vi "5492_Get_YPRHfH.vi"(5 "Device Number":T1, 7 "Update":bool, 8 "error in":errorcluster) -> (0 "error out":errorcluster, 2 "YRPHfH":T2)   [LabVIEW 2016]
doc: "This navX VI returns the Yaw, Roll, Pitch, Heading, Fused Heading of the navX."
uses:
  <vilib>/Rock Robotics/WPI/ThirdParty/Sensors/navX/_TypeDefs/FRIC_navX_DeviceNumbersTypeDef.ctl
  <vilib>/Rock Robotics/WPI/ThirdParty/Sensors/navX/_TypeDefs/Z900_navX_DeviceRegisters.ctl
  <vilib>/Rock Robotics/WPI/ThirdParty/Sensors/navX/_Util/Z900_navX_Util_LittleEndian_to_BigEndian.vi
  <vilib>/Rock Robotics/WPI/ThirdParty/Sensors/navX/Get/_Internal/FRIC_navX_Get_Registry.vi
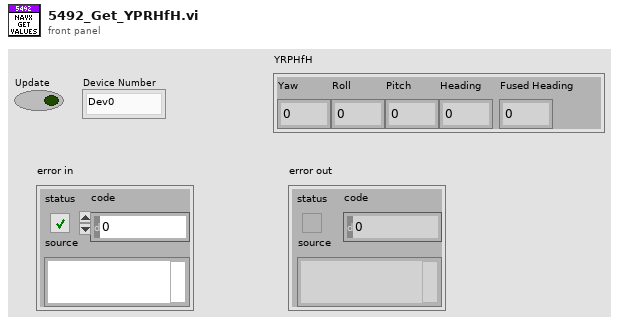
[diagram p1: front panel]
types:
  T1 = typedef "FRIC_navX_DeviceNumbersTypeDef.ctl" = enum16{"Dev0", "Dev1", "Dev2", "Dev3"}
  T2 = cluster{"Yaw":dbl, "Roll":dbl, "Pitch":dbl, "Heading":dbl, "Fused Heading":dbl}
  T3 = typedef "Z900_navX_DeviceRegisters.ctl" = u8
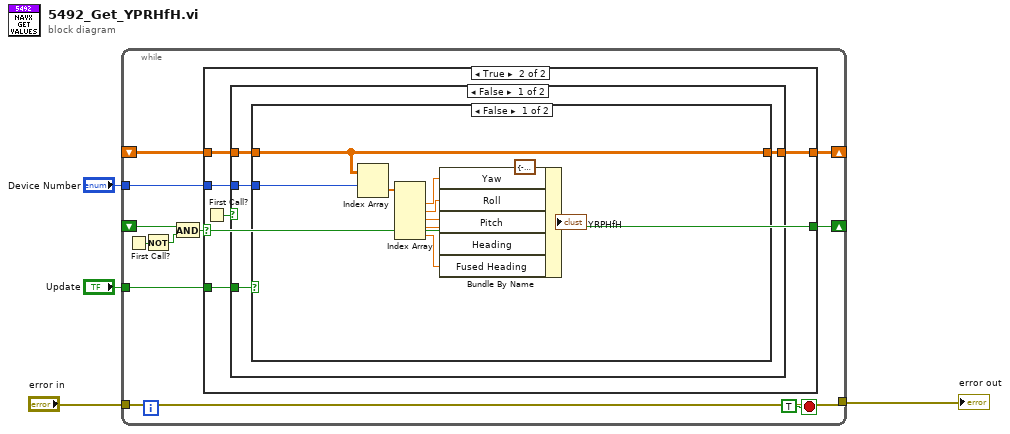
[diagram p0: block diagram]
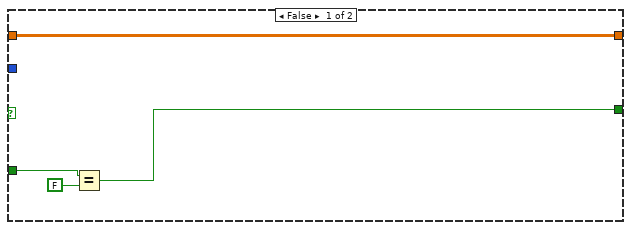
[diagram p2: hidden frame]
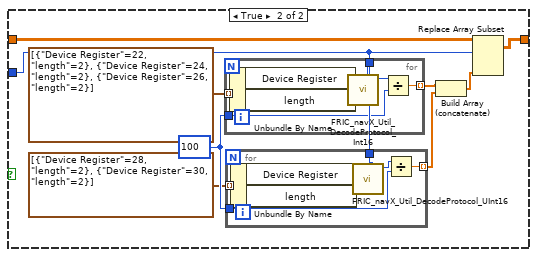
[diagram p3: hidden frame]
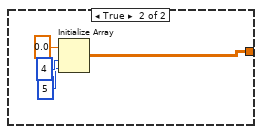
[diagram p4: hidden frame]
diagram:
  n1 = while {
    shift-right: [w13] -> _
    shift-left: _ -> [w14]
    tunnel: "Update" -> [w12]
    tunnel: "Device Number" -> [w11]
    shift-right: [w10] -> _
    shift-left: _ -> [w9]
    tunnel: "error in" -> [w5]
    tunnel: [w5] -> w1
    stop <- TRUE stop-if-true
    n2 = First Call?() -> (First Call?: T/F=w8:bool)
    n3 = Not(x=w8) -> (.not. x?=w7:bool)
    n4 = And(x=w9, y=w7) -> (x .and. y?=w6:bool)
    n5 = case shown="True" w6 {
      selector: w6 -> [_ w20]
      tunnel: w14 -> [w19 w25]
      tunnel: [w19 w24] -> w13
      tunnel: w12 -> [w18 w23]
      tunnel: w11 -> [_ w22]
      tunnel: [w16 w20] -> w10
      frame False {
        n6 = Equal?(x=w18, y=FALSE) -> (x = y?=w16:bool)
      }
      frame True {
        n7 = First Call?() -> (First Call?: T/F=w21:bool)
        n8 = case shown="False" w21 {
          tunnel: w25 -> [w29 _]
          tunnel: [w28 w66] -> w24
          tunnel: w23 -> [w26 _]
          tunnel: w22 -> [w27 _]
          frame False {
            n9 = case shown="False" w26 {
              tunnel: [w39 w46] -> w28
              tunnel: w29 -> [w39 w48]
              tunnel: w27 -> [w38 w47]
              frame False {
                n10 = Index Array(array=w39, index (row)=w38) -> (element=w35:dbl[])  [unwired: 1 in]
                n11 = Index Array(array=w35) -> (element #1=w34:dbl, element #2=w33:dbl, element #3=w32:dbl, element #4=w31:dbl, element #5=w30:dbl)  [unwired: 5 in]
                n12 = Bundle By Name(cluster=T2 {"Yaw"=-0.34, "Roll"=0.2, "Pitch"=0.2, "Heading"=0.0, "Fused Heading"=359.65} ("YRPHfH"), "Yaw"=w34, "Roll"=w33, "Pitch"=w32, "Heading"=w31, "Fused Heading"=w30) -> (→"YRPHfH":T2)
              }
              frame True {
                w44 = 100 ("y")
                n13 = for {
                  tunnel: w47 -> [w54]
                  tunnel: cluster{"Device Register":T3, "length":i32}[] [{"Device Register"=22, "length"=2}, {"Device Register"=24, "length"=2}, {"Device Register"=26, "length"=2}] ("Array") -> [w53] mode=indexing
                  tunnel: w44 -> [w50]
                  tunnel: [w49] -> w42 mode=indexing
                  n14 = Unbundle By Name(w53) -> ("Device Register"=w52:T3, "length"=w55:i32)
                  n15 = call <vilib>:"FRIC_navX_Util_DecodeProtocol_Int16.vi"("Device Number"=w54, "length"=w55, "Device Register"=w52) -> ("Value"=w51:i16)  [unwired: 8 in]
                  n16 = Divide(x=w51, y=w50) -> (x/y=w49:dbl)
                }
                n17 = for {
                  tunnel: cluster{"Device Register":T3, "length":i32}[] [{"Device Register"=28, "length"=2}, {"Device Register"=30, "length"=2}] ("Array") -> [w62] mode=indexing
                  tunnel: w47 -> [w59]
                  tunnel: w44 -> [w57]
                  tunnel: [w56] -> w41 mode=indexing
                  n18 = Unbundle By Name(w62) -> ("Device Register"=w61:T3, "length"=w60:i32)
                  n19 = call <vilib>:"FRIC_navX_Util_DecodeProtocol_UInt16.vi"("Device Number"=w59, "length"=w60, "Device Register"=w61) -> ("Value"=w58:u16)  [unwired: 8 in]
                  n20 = Divide(x=w58, y=w57) -> (x/y=w56:dbl)
                }
                n21 = Build Array (concatenate)(w42, w41) -> (w40:dbl[])
                n22 = Replace Array Subset(array=w48, new element=w40, index (row)=w47) -> (w46:dbl[][])  [unwired: 1 in]
              }
            }
          }
          frame True {
            n23 = Initialize Array(0.0, 4, 5 ("dimension size")) -> (w66:dbl[][])
          }
        }
      }
    }
  }
  "error out" <- w1
